vi "ZCAN_InitCAN(EU).vi"(0 "device_hande":u32, 5 "can_index":u32, 7 "ZCAN_InitCAN_Setting_EU":T1, 11 "error in (no error)":errorcluster caption="错误输入（无错误）") -> (8 "can_index_handle":u32, 15 "error out":errorcluster caption="错误输出")   [LabVIEW 2018]
doc: "用于设置CAN通道的初始化参数。\n\n适用的设备：PCI-5010-U、PCI-5020-U、USBCAN-E-U、USBCAN-2E-U、CANalyst-II+"
uses:
  zlgcan_labview_20220510/zlgcan_demo_EU/bin/zlgcan_wrap.dll
  data_type/ZCAN_InitCAN_setting_EU.ctl
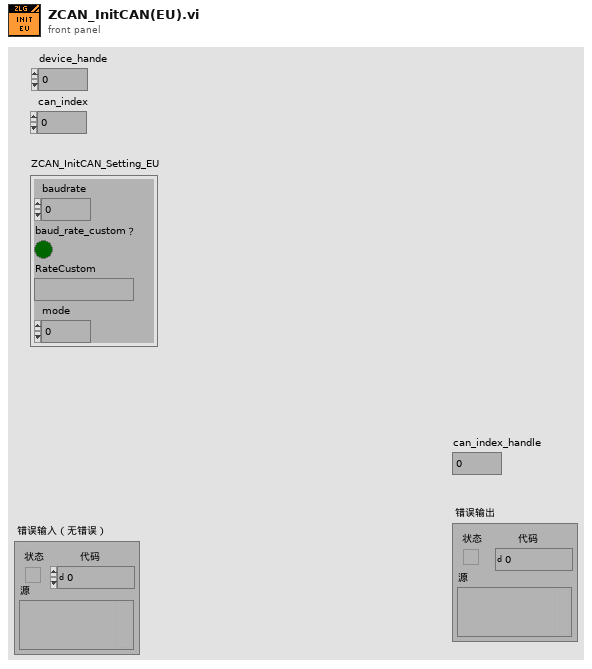
[diagram p1: front panel]
types:
  T1 = typedef "ZCAN_InitCAN_setting_EU.ctl" = cluster{"baudrate":u32, "baud_rate_custom？":bool, "RateCustom":string, "mode":u8}
  T2 = cluster{"can_type":u32, "can_type":u32, "can_type":u32, "can_type":u32, "can_type":u8, "can_type":u8, "can_type":u8, "mode":u8}
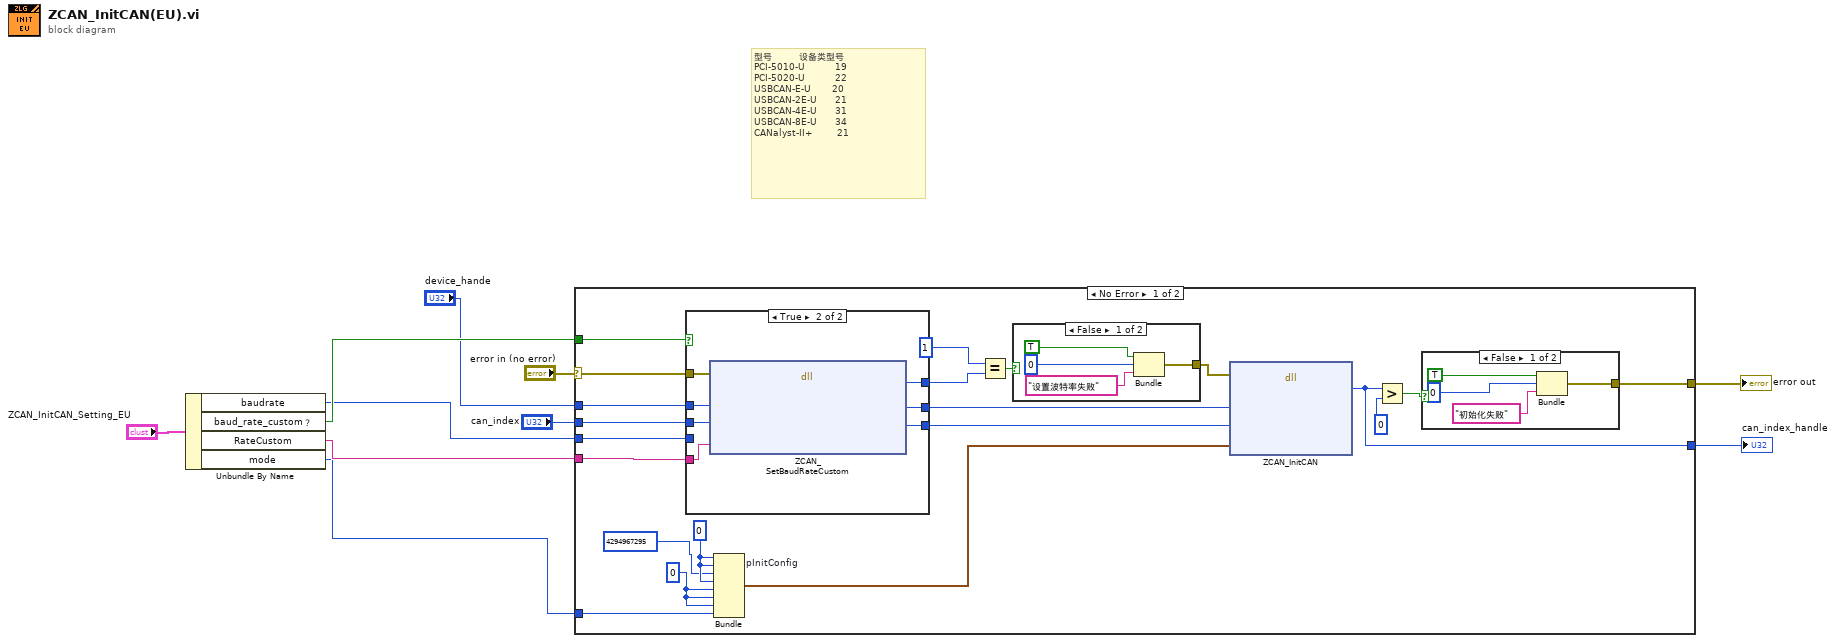
[diagram p0: block diagram]
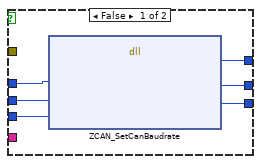
[diagram p4: hidden frame]
diagram:
  # "型号         设备类型号\nPCI-5010-U          19 \nPCI-5020-U          22\nUSBCAN-E-U       20\nUSBCAN-2E-U      21\nUSBCAN-4E-U      31\nUSBCAN-8E-U      34\nCANalyst-II+        21"
  n1 = Unbundle By Name("ZCAN_InitCAN_Setting_EU") -> ("baudrate"=w3:u32, "baud_rate_custom？"=w5:bool, "RateCustom"=w2:string, "mode"=w1:u8)
  n2 = case shown="No Error" "error in (no error)" {
    selector: "error in (no error)" -> [w25 w53]
    tunnel: [w24 w53] -> w9
    tunnel: w5 -> [w31 _]
    tunnel: "device_hande" -> [w30 _]
    tunnel: "can_index" -> [w29 _]
    tunnel: w3 -> [w28 _]
    tunnel: w2 -> [w27 _]
    tunnel: w1 -> [w26 _]
    tunnel: [w23 _] -> w7
    frame No Error {
      w13 = u8 0 ("can_type")
      w14 = u32 0 ("can_type")
      n3 = case shown="True" w31 {
        tunnel: [w44 w52] -> w22
        tunnel: [w43 w51] -> w21
        tunnel: [w45 w50] -> w19
        tunnel: w30 -> [w42 w48]
        tunnel: w29 -> [w41 w47]
        tunnel: w28 -> [w40 _]
        tunnel: w27 -> [_ w49]
        tunnel: w25 -> [_ w46]
        frame False {
          n4 = dll-call lib="C:/Users/admin/Desktop/zlgcan_labview_20220510/zlgcan_demo_EU/bin/zlgcan_wrap.dll" fn="ZCAN_SetCanBaudrate"("hDev"=w42, "can_index"=w41, "baudrate"=w40) -> ("return"=w45:u32, "hDev"=w44:u32, "can_index"=w43:u32)  [unwired: 4 in, 2 out]
        }
        frame True {
          n5 = dll-call lib="C:/Users/admin/Desktop/zlgcan_labview_20220510/zlgcan_demo_EU/bin/zlgcan_wrap.dll" fn="ZCAN_SetBaudRateCustom"(error in=w46, "device_handle"=w48, "can_index"=w47, "RateCustom"=w49) -> ("return"=w50:u32, "device_handle"=w52:u32, "can_index"=w51:u32)  [unwired: 3 in, 2 out]
        }
      }
      n6 = Bundle "pInitConfig"("can_type"=w14, "can_type"=w14, "can_type"=u32 4294967295, "can_type"=w14, "can_type"=w13, "can_type"=w13, "can_type"=w13, "mode"=w26) -> (w12:T2)  [unwired: 1 in]
      n7 = Equal?(x=1, y=w19) -> (x = y?=w18:bool)
      n8 = case shown="False" w18 {
        tunnel: [w36 _] -> w17
        frame False {
          n9 = Bundle("status"=TRUE, "code"=0, "消息"="设置波特率失败") -> (w36:cluster{"status":bool, "code":i32, "消息":string})  [unwired: 1 in]
        }
        frame True {
        }
      }
      n10 = dll-call lib="C:/Users/admin/Desktop/zlgcan_labview_20220510/zlgcan_demo_EU/bin/zlgcan_wrap.dll" fn="ZCAN_InitCAN"(error in=w17, "device_handle"=w22, "can_index"=w21, "pInitConfig"=w12) -> ("can_handle"=w23:u32)  [unwired: 5 in, 2 out]
      n11 = Greater?(x=w23, y=0) -> (0:w15:bool)
      n12 = case shown="False" w15 {
        tunnel: [w32 _] -> w24
        frame False {
          n13 = Bundle("status"=TRUE, "code"=0, "消息"="初始化失败") -> (w32:cluster{"status":bool, "code":i32, "消息":string})  [unwired: 1 in]
        }
        frame True {
        }
      }
    }
    frame Error {
    }
  }
  "error out" <- w9
  "can_index_handle" <- w7
